vi "ITC503 read A.vi"(8 "error in (no error)":errorcluster, 9 "Sensor #":i32=1, 11 "VISA resource name":refnum<visa-resource-name>) -> (0 "error out":errorcluster, 1 "read buffer":string, 2 "Temperature":dbl, 3 "VISA resource name out":refnum<visa-resource-name>)   [LabVIEW 2010]
panel:
  in  "Address":refnum<visa-resource-name>
  in  "Command":string
  out "Reply":string="ITC503 Version 1.11 (c) OXFORD 1997\r"
  out "Numeric reply":dbl format="%.2f"
  out "error out 2":errorcluster
  in  "error in (no error) 2":errorcluster
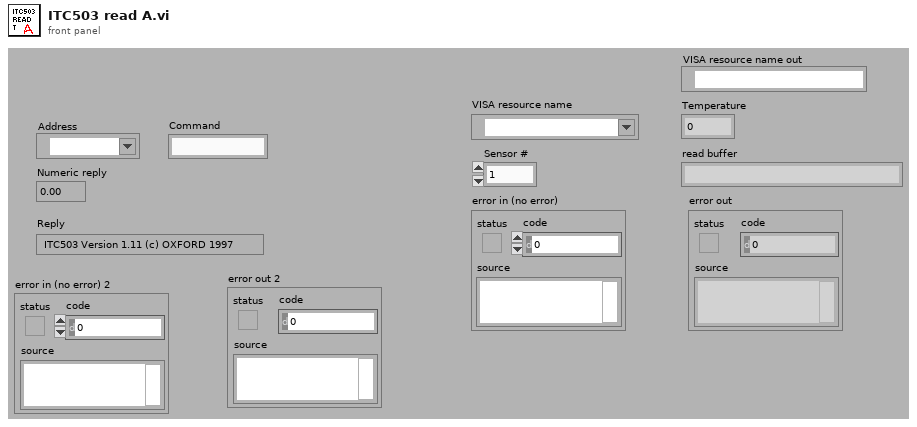
[diagram p1: front panel]
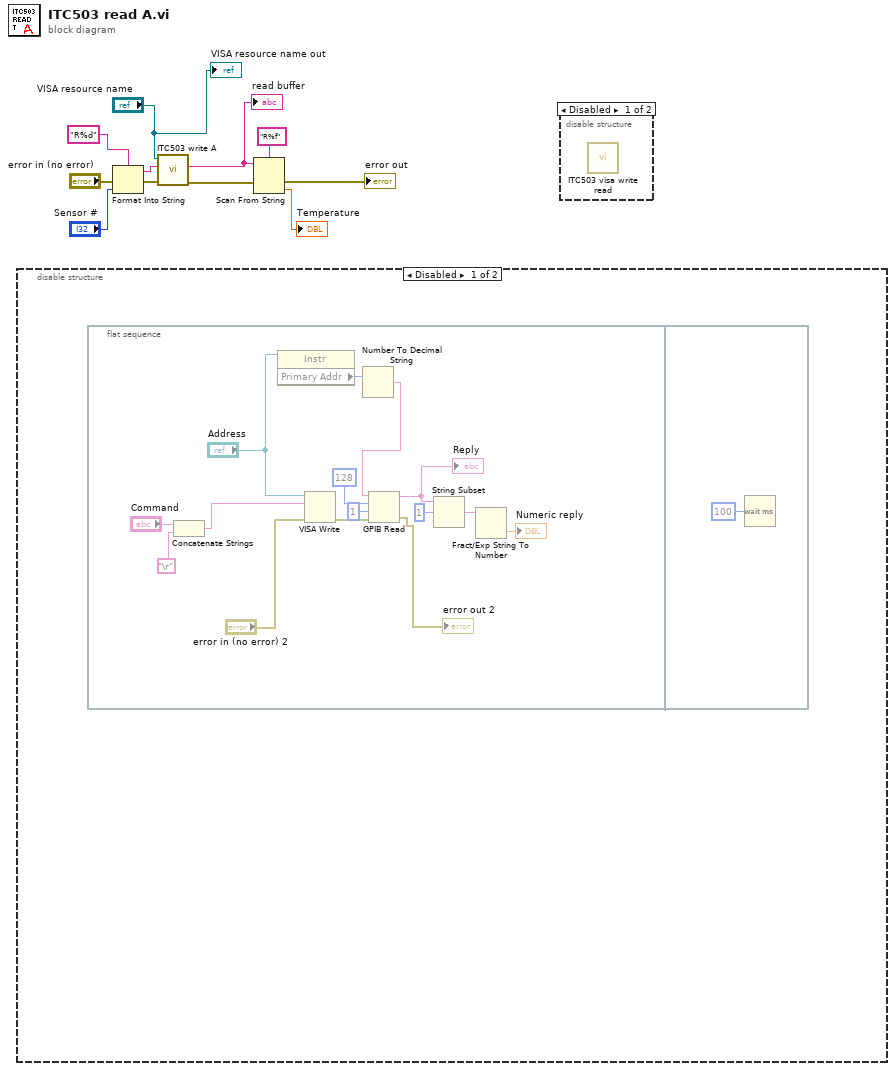
[diagram p0: block diagram]
diagram:
  n1 = disable-structure shown="Disabled" {
    frame Disabled {
      n2 = flat-sequence {
        frame #0 {
          n3 = Concatenate Strings("Command", "\r") -> (w25:string)
          n4 = property class="Instr"(reference="Address") -> ("Primary Addr"=w18:u16)  [unwired: 1 in, 2 out]
          n5 = VISA Write(VISA resource name="Address", write buffer=w25, error in (no error)="error in (no error) 2") -> (error out=w17:errorcluster)  [unwired: 2 out]
          n6 = Number To Decimal String(number=w18) -> (decimal integer string=w15:string)  [unwired: 1 in]
          n7 = GPIB Read(0:w15, 1:u32 128 ("byte count"), 2:i16 1 ("mode (0)"), 3:w17) -> (5:w12:string, 7:→"error out 2":errorcluster)  [unwired: 1 in, 1 out]
          "Reply" <- w12
          n8 = String Subset(string=w12, offset (0)=1) -> (substring=w22:string)  [unwired: 1 out]
          n9 = Fract/Exp String To Number(string=w22) -> (number=→"Numeric reply":dbl)  [unwired: 4 out]
        }
        frame #1 {
          n10 = Wait (ms)(milliseconds to wait=u32 100) -> ()  [unwired: 1 out]
        }
      }
    }
    frame Enabled {
    }
  }
  n11 = Format Into String(format string="R%d" ("write buffer"), error in="error in (no error)", "Sensor #") -> (resulting string=w5:string, error out=w6:errorcluster)  [unwired: 1 in]
  n12 = call "ITC503 write A.vi"("error in (no error) 2"=w6, "write buffer 2"=w5, "VISA resource name 2"="VISA resource name") -> ("error out 2"=w2:errorcluster, "read buffer 2"=w4:string)  [unwired: 5 in, 2 out]
  "read buffer" <- w4
  n13 = Scan From String(format string="R%f", input string=w4, error in=w2) -> (error out=→"error out":errorcluster, output 1=→"Temperature":dbl)  [unwired: 2 in, 2 out]
  n14 = disable-structure shown="Disabled" {
    frame Disabled {
      n15 = call "ITC503 visa write read.vi"() -> ()  [unwired: 9 in, 3 out]
    }
    frame Enabled {
    }
  }
  "VISA resource name out" <- "VISA resource name"
